vi "Define 2D Heat PDE IC (Numeric).vi"(0 "PDE in":refnum<class "NI_PDE.lvclass">, 5 "Initial Condition":dbl[][](array[numeric]), 11 "error in (no error)":errorcluster) -> (4 "PDE out":refnum<class "NI_PDE.lvclass">, 15 "error out":errorcluster)   [LabVIEW 2020, in "NI_PDE.lvlib"]
doc: "Defines the initial condition of a partial differential equation. You must manually select the polymorphic instance to use."
uses:
  <vilib>/gmath/NI_PDE.lvlib
  <vilib>/gmath/pde.llb/PDEClass/NI_PDE.lvclass
  <vilib>/gmath/pde.llb/PDEClass/PDE_Heat_2D/NI_PDE_Heat_2D.lvclass
  e:/builds/penguin/labview/branches/2020/dev/dist/vi.lib/gmath/pde.llb/PDEClass/NI_PDE.lvclass
  <vilib>/gmath/pde.llb/Common/PDE_IC Type.ctl
  <vilib>/gmath/pde.llb/ICClass/IC_2D_Numeric/NI_IC_2D_Numeric.lvclass
  e:/builds/penguin/labview/branches/2020/dev/dist/vi.lib/gmath/pde.llb/ICClass/NI_IC.lvclass
  <vilib>/gmath/pde.llb/ICClass/IC_2D_Numeric/IC Data.ctl
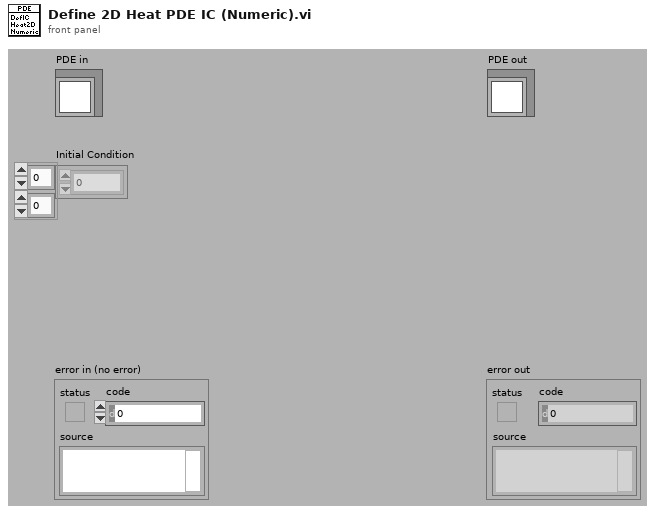
[diagram p1: front panel]
types:
  T1 = typedef "NI_PDE.lvlib/PDE_IC Type.ctl" = i32
  T2 = typedef "NI_PDE.lvlib/NI_IC_2D_Numeric.lvclass/IC Data.ctl" = cluster{"type":T1, "H":dbl[][]}
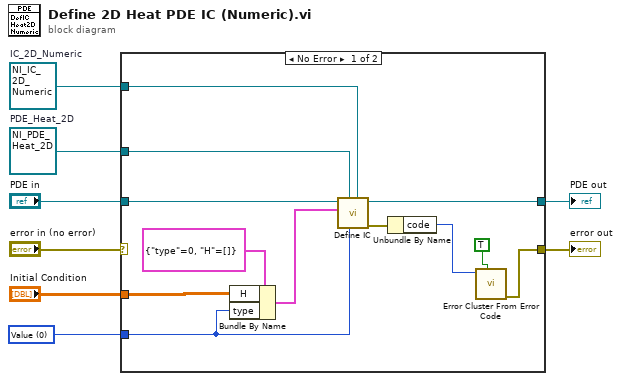
[diagram p0: block diagram]
diagram:
  w1 = refnum<class "NI_IC_2D_Numeric.lvclass"> refnum  # IC_2D_Numeric
  w3 = T1 0 items=["Value", "Derivative"] ("type")
  w2 = refnum<class "NI_PDE_Heat_2D.lvclass"> refnum  # PDE_Heat_2D
  n1 = case shown="No Error" "error in (no error)" {
    selector: "error in (no error)" -> [_ w21]
    tunnel: "PDE in" -> [w9 w22]
    tunnel: [w15 w22] -> w7
    tunnel: "Initial Condition" -> [w13 _]
    tunnel: [w18 w21] -> w5
    tunnel: w3 -> [w12 _]
    tunnel: w2 -> [w11 _]
    tunnel: w1 -> [w10 _]
    frame No Error {
      n2 = Bundle By Name(cluster=T2 {"type"=0, "H"=[]} ("IC data"), "H"=w13, "type"=w12) -> (w16:T2)
      n3 = call <vilib>:"Define IC.vi"("target IC"=w10, "index"=w12, "target PDE"=w11, "IC"=w16, "PDE in"=w9) -> ("error out"=w14:errorcluster, "PDE out"=w15:refnum<class "NI_PDE.lvclass">)  [unwired: 2 in, 3 out]
      n4 = Unbundle By Name(w14) -> ("code"=w20:i32)
      n5 = call <vilib>:"Error Cluster From Error Code.vi"("show call chain? (False)"=TRUE, "error code (0)"=w20) -> ("error out"=w18:errorcluster)  [unwired: 1 in, 6 out]
    }
    frame Error {
    }
  }
  "PDE out" <- w7
  "error out" <- w5
